vi "Ejercicio_18_derecha_izquierda.vi"() -> ()   [LabVIEW 2020]
uses:
  <vilib>/Instr/_visa.llb/VISA Configure Serial Port (Instr).vi
panel:
  in  "Configuacion UART":T1={"Puerto"="", "baud rate (9600)"=9600, "parity (0:none)"=enum."None", "data bits (8)"=8} {"data bits (8)" min=5 max=8 step=1}
  in  "stop":bool
  in  "Duty Cycle (%)":dbl=50.0
  out "Waveform Graph":dynamicdata(graph)
  out "Datos recibidos":string
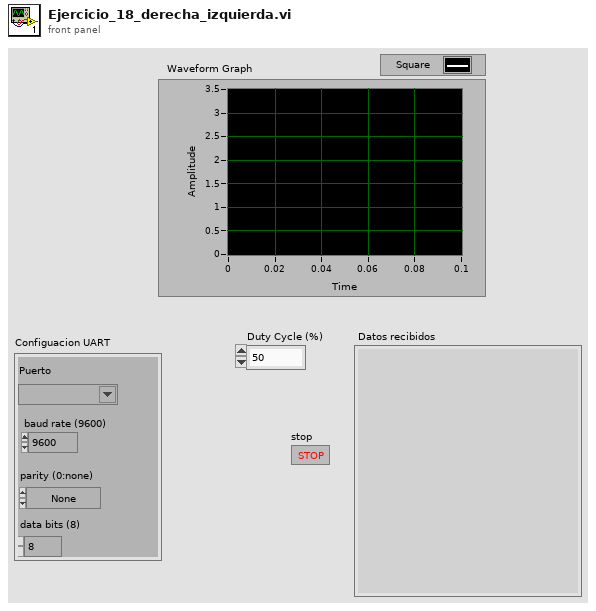
[diagram p1: front panel]
types:
  T1 = cluster{"Puerto":refnum<visa-resource-name>, "baud rate (9600)":u32, "parity (0:none)":enum16{"None", "Odd", "Even", "Mark", "Space"}, "data bits (8)":u16}
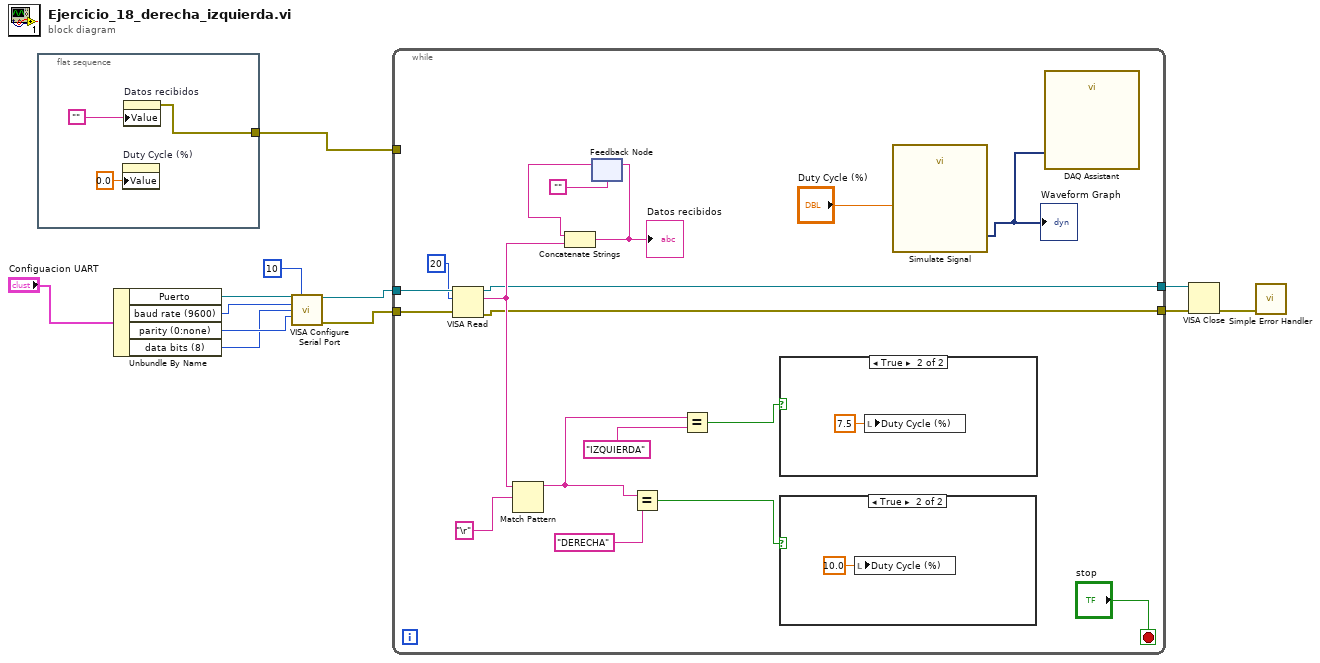
[diagram p0: block diagram]
diagram:
  n1 = flat-sequence {
    tunnel: [w13] -> w8
    frame #0 {
      n2 = property on="Duty Cycle (%)" class="DigNum (strict)"("Value"=0.0 ("Duty Cycle (%)")) -> ()  [unwired: 2 in, 2 out]
      n3 = property on="Datos recibidos" class="Str"("Value"="") -> (error out=w13:errorcluster)  [unwired: 2 in, 1 out]
    }
  }
  n4 = Unbundle By Name("Configuacion UART") -> ("Puerto"=w6:refnum<visa-resource-name>, "baud rate (9600)"=w5:u32, "parity (0:none)"=w4:enum16{"None", "Odd", "Even", "Mark", "Space"}, "data bits (8)"=w3:u16)
  n5 = call-poly "VISA Configure Serial Port"("VISA resource name"=w6, "timeout (10sec)"=u32 10, "baud rate (9600)"=w5, "data bits (8)"=w3, "parity (0:none)"=w4) -> ("VISA resource name out"=w12:refnum<visa-resource-name>, "error out"=w11:errorcluster)  [unwired: 9 in]
  n6 = while {
    tunnel: w12 -> [w27]
    tunnel: w11 -> [w26]
    tunnel: [w19] -> w10
    tunnel: [w17] -> w9
    tunnel: w8 -> [_]
    stop <- "stop" stop-if-true
    n7 = VISA Read(VISA resource name=w27, byte count=u32 20, error in (no error)=w26) -> (VISA resource name out=w17:refnum<visa-resource-name>, read buffer=w24:string, error out=w19:errorcluster)  [unwired: 1 out]
    n8 = Match Pattern(string=w24, regular expression="\r") -> (before substring=w30:string)  [unwired: 1 in, 3 out]
    n9 = feedback #1("") -> (w18:string)
    n10 = Concatenate Strings(w18, w24) -> (w23:string)
    "Datos recibidos" <- w23
    n11 = feedback-in #1(w23) -> ()
    n12 = Equal?(x=w30, y="DERECHA") -> (x = y?=w20:bool)
    n13 = Equal?(x=w30, y="IZQUIERDA") -> (x = y?=w21:bool)
    n14 = case shown="True" w21 {
      frame False {
      }
      frame True {
        n15 = local write "Duty Cycle (%)"(7.5 ("Duty Cycle (%)")) -> ()
      }
    }
    n16 = case shown="True" w20 {
      frame False {
      }
      frame True {
        n17 = local write "Duty Cycle (%)"(10.0 ("Duty Cycle (%)")) -> ()
      }
    }
    n18 = call "Simulate Signal"("Duty Cycle (%)"="Duty Cycle (%)") -> ("Square"=w16:dynamicdata)  [unwired: 13 in, 1 out]
    "Waveform Graph" <- w16
    n19 = call "DAQ Assistant"("data"=w16) -> ()  [unwired: 16 in, 3 out]
  }
  n20 = VISA Close(VISA resource name=w9, error in (no error)=w10) -> (error out=w1:errorcluster)
  n21 = call <vilib>:"Simple Error Handler.vi"("error in (no error)"=w1) -> ()  [unwired: 4 in, 5 out]
